vi "example of controlling MC remotely.vi"() -> ()   [LabVIEW 2020]
panel:
  in  "command":string="ScanStart"
  out "data out":string
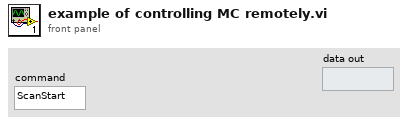
[diagram p1: front panel]
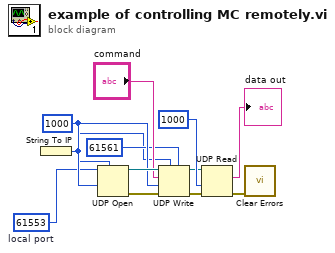
[diagram p0: block diagram]
diagram:
  w1 = u16 61553  # local port
  w10 = 1000 ("timeout ms (25000)")
  n1 = String To IP() -> (0:w2:u32)  [unwired: 1 in]
  n2 = UDP Open(7:w2, 9:w10, 11:w1) -> (port=w11:refnum<k16>, 0:w12:errorcluster)  [unwired: 2 in, 1 out]
  n3 = UDP Write(address=w2, port or service name=u16 61561 ("port"), connection ID=w11, data in="command", 8:w12, 9:w10) -> (error out=w7:errorcluster, 3:w8:refnum<k16>)
  n4 = UDP Read(connection ID=w8, timeout ms (25000)=1000, 8:w7) -> (data out=→"data out":string, error out=w6:errorcluster)  [unwired: 1 in, 3 out]
  n5 = call <vilib>:"Clear Errors.vi"("error in (no error)"=w6) -> ()  [unwired: 5 in, 2 out]
